vi "get range of comic last_updates.vi"() -> ()   [LabVIEW 2024]
uses:
  CV_RESTful_Library/typedefs/cv_date_updated.results--array.ctl
  <vilib>/addons/_JKI.lib/REST Client/classes/REST Client/REST Client.lvclass
  CV_RESTful_Library/CV_RESTful_Lib.lvlib
panel:
  out "results":T1
  in  "volume id":i32
  out "error out":errorcluster
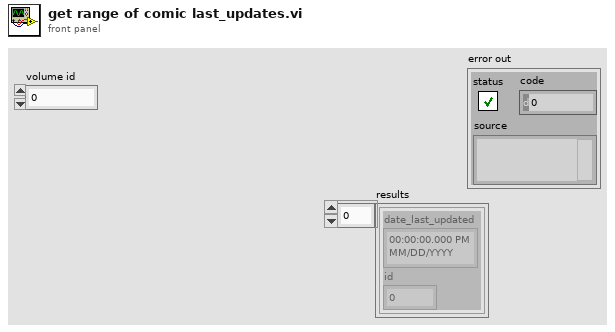
[diagram p1: front panel]
types:
  T1 = typedef "CV_RESTful_Lib.lvlib/cv_date_updated.results--array.ctl" = cluster{"date_last_updated":timestamp, "id":i32}[]
  T2 = typedef "cv_date_updated.results--array.ctl" = cluster{"date_last_updated":timestamp, "id":i32}[]
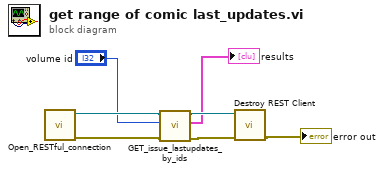
[diagram p0: block diagram]
diagram:
  n1 = call "Open_RESTful_connection.vi"() -> ("error out"=w5:errorcluster, "REST Client out"=w6:refnum<class "REST Client.lvclass">)  [unwired: 10 in]
  n2 = call "GET_issue_lastupdates_by_ids.vi"("error in (no error)"=w5, "volume id"="volume id", "REST Client in"=w6) -> ("error out"=w4:errorcluster, "results"=→"results":T2, "REST Client out"=w3:refnum<class "REST Client.lvclass">)  [unwired: 6 in]
  n3 = call-dynamic "Destroy REST Client.vi"("error in (no error)"=w4, "REST Client in"=w3) -> ("error out"=→"error out":errorcluster)  [unwired: 9 in]
